vi "Read Motor Obj.vi"(8 "error in (no error)":errorcluster, 11 "Motor Configuration in":refnum<class "Motor Configuration.lvclass">) -> (0 "error out":errorcluster, 2 "Hardware.lvlib:Motor.lvlib:Motor.lvclass":refnum<class "Motor.lvclass">, 3 "Motor Configuration out":refnum<class "Motor Configuration.lvclass">)   [LabVIEW 2016, in "Hardware.lvlib" / "Motor.lvlib" / "Motor Configuration.lvclass"]
uses:
  <userlib>/Common Components/Hardware/Motor/Motor Config/Motor Configuration.lvclass
  <userlib>/Common Components/Hardware/Motor/Motor/Motor.lvclass
  <userlib>/Common Components/Hardware/Motor/Motor Config/Motor Configuration.lvclass/Motor Configuration.ctl
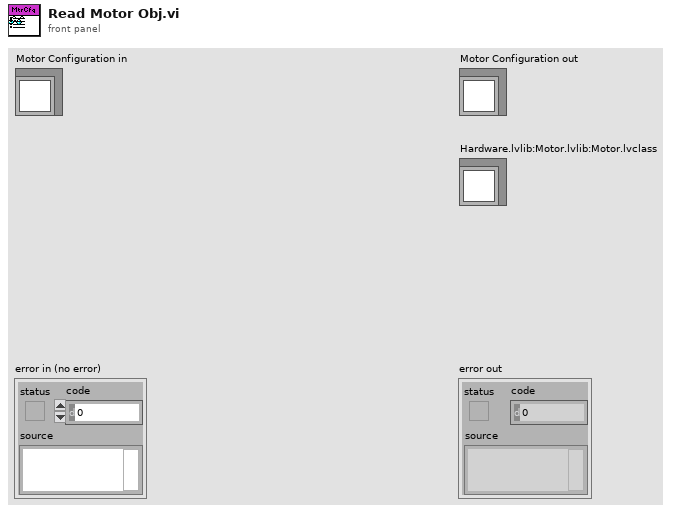
[diagram p1: front panel]
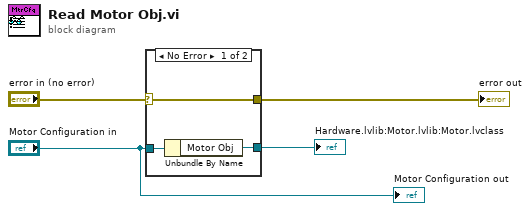
[diagram p0: block diagram]
diagram:
  n1 = case shown="No Error" "error in (no error)" {
    selector: "error in (no error)" -> [w5 w8]
    tunnel: "Motor Configuration in" -> [w7 _]
    tunnel: [w6 _] -> w3
    tunnel: [w5 w8] -> w1
    frame No Error {
      n2 = Unbundle By Name(w7) -> ("Motor Obj"=w6:refnum<class "Motor.lvclass">)
    }
    frame Error {
    }
  }
  "error out" <- w1
  "Hardware.lvlib:Motor.lvlib:Motor.lvclass" <- w3
  "Motor Configuration out" <- "Motor Configuration in"
